vi "SimpleExportUseBookmark.vi"(4 "GraphBookmark":string, 5 "StringData":string[](array[string]), 6 "GraphReference":refnum<vi>, 7 "BookmarkTarget":string[](array[string]), 8 "error in (no error)":errorcluster, 10 "TemplateFilePath":path) -> (0 "error out":errorcluster)   [LabVIEW 8.6]
uses:
  <vilib>/Utility/NIReport.llb/NI_report.lvclass
  <vilib>/Utility/NIReport.llb/Append Report Text (str wrap).vi
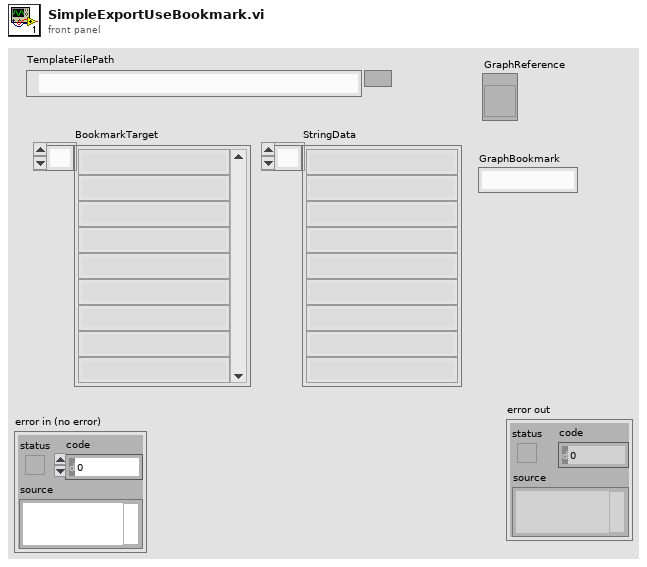
[diagram p1: front panel]
types:
  T1 = cluster{"position (excel)":cluster{"row":i32, "column":i32}, "name (excel)":string, "bookmark (word)":string}
  T2 = enum16{"Standard Report", "HTML", "Word", "Excel"}
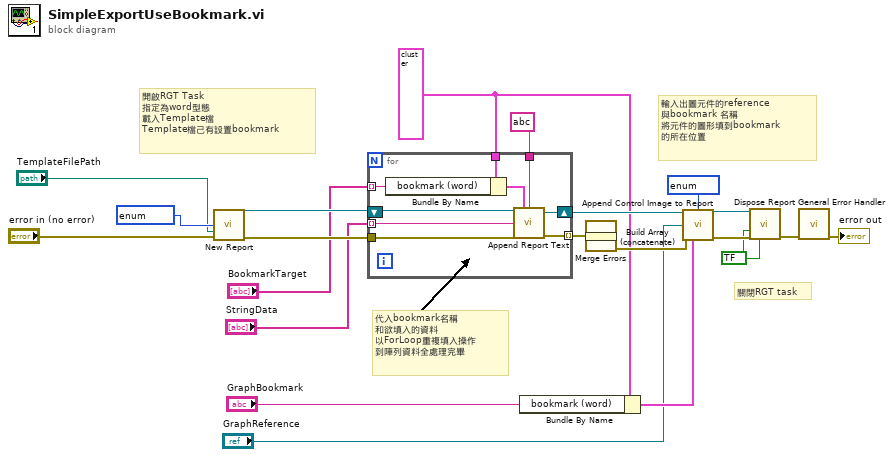
[diagram p0: block diagram]
diagram:
  w6 = bool ? ("save changes? (F)")
  w11 = T1 ? ("MS Office parameters")
  # "關閉RGT task"
  # "輸入出圖元件的reference\n與bookmark 名稱\n將元件的圖形填到bookmark\n的所在位置"
  # "代入bookmark名稱\n和欲填入的資料\n以ForLoop重複填入操作\n到陣列資料全處理完畢"
  # "開啟RGT Task\n指定為word型態\n載入Template檔\nTemplate檔己有設置bookmark"
  n1 = call <vilib>:"New Report.vi"("report type"=T2 ?, "template (empty)"="TemplateFilePath", "error in (no error)"="error in (no error)") -> ("report out"=w20:refnum<class "NI_report.lvclass">, "error out"=w19:errorcluster)  [unwired: 11 in]
  n2 = for {
    tunnel: w11 -> [w31]
    tunnel: w19 -> [w28]
    tunnel: "BookmarkTarget" -> [w27] mode=indexing
    tunnel: "StringData" -> [w26] mode=indexing
    tunnel: string ? ("format string (%.3f)") -> [w25]
    shift-right: [w24] -> w15
    shift-left: w20 -> [w29]
    tunnel: [w23] -> w14 mode=indexing
    n3 = Bundle By Name(cluster=w31, "bookmark (word)"=w27) -> (w30:T1)
    n4 = call-poly <vilib>:"Append Report Text.vi"("report in"=w29, "MS Office parameters"=w30, "format string (%.3f)"=w25, "text"=w26, "error in (no error)"=w28) -> ("report out"=w24:refnum<class "NI_report.lvclass">, "error out"=w23:errorcluster)  [unwired: 7 in, 2 out]
  }
  n5 = Bundle By Name(cluster=w11, "bookmark (word)"="GraphBookmark") -> (w9:T1)
  n6 = Build Array (concatenate)(w14) -> (w1:errorcluster[])
  n7 = call <vilib>:"Merge Errors.vi"("error array in"=w1) -> ("error out"=w13:errorcluster)  [unwired: 6 in]
  n8 = call-dynamic "Append Control Image to Report.vi"("report in"=w15, "image file type (.jpg)"=enum16{".jpg", ".png"} ?, "ctrl reference"="GraphReference", "error in (no error)"=w13, "MS Office parameters"=w9) -> ("report out"=w8:refnum<class "NI_report.lvclass">, "error out"=w7:errorcluster)  [unwired: 7 in, 2 out]
  n9 = call-dynamic "Dispose Report.vi"("report in"=w8, "save changes? (F)"=w6, "error in (no error)"=w7, "close report? (T)"=w6) -> ("error out"=w5:errorcluster)  [unwired: 11 in]
  n10 = call <vilib>:"General Error Handler.vi"("error in (no error)"=w5) -> ("error out"=→"error out":errorcluster)  [unwired: 10 in, 4 out]
